vi "日志信息主动发送(子VI).vi"(10 "是否正在查询数据":bool, 11 "查询数据发送时间节点":string) -> ()   [LabVIEW 2016, in "数据传输系统.lvlib"]
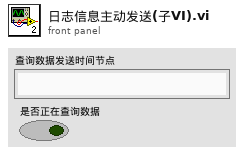
[diagram p1: front panel]
types:
  T1 = typedef "LVDateTimeRec.ctl" = cluster{"秒数的小数部分":dbl, "秒":i32, "分":i32, "时":i32, "日":i32, "月":i32, "年":i32, "天数（周）":i32, "天数（年）":i32, "DST":i32}
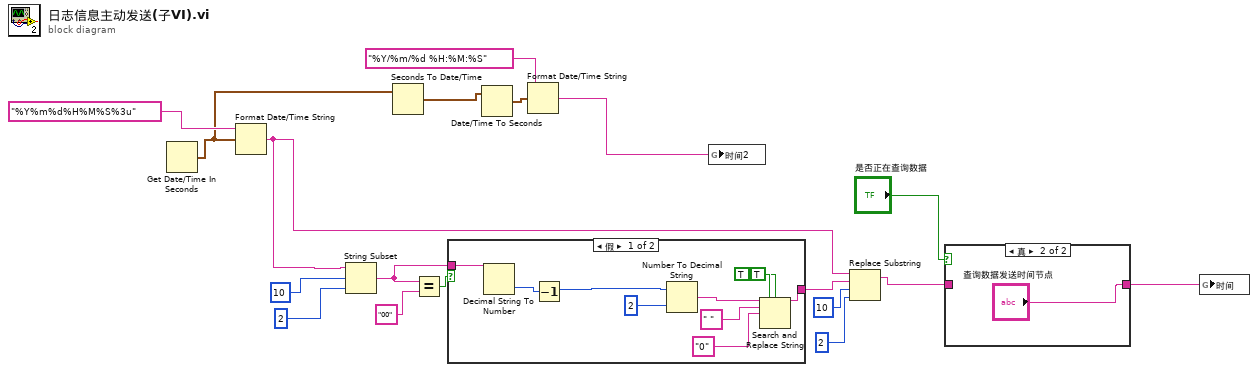
[diagram p0: block diagram]
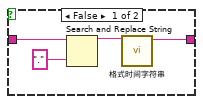
[diagram p2: hidden frame]
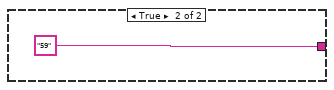
[diagram p3: hidden frame]
diagram:
  n1 = Get Date/Time In Seconds() -> (seconds since 1Jan1904=w2:timestamp)
  n2 = Format Date/Time String(time format string (%c)="%Y%m%d%H%M%S%3u" ("时间格式字符串(%c)"), seconds (now)=w2) -> (date/time string=w7:string)  [unwired: 1 in]
  n3 = String Subset(string=w7, offset (0)=10 ("偏移量(0)"), length (rest)=2 ("长度（子字符串长度）")) -> (substring=w15:string)
  n4 = Seconds To Date/Time(time stamp (now)=w2) -> (date time rec=w3:T1)  [unwired: 1 in]
  n5 = Equal?(x=w15, y="00") -> (x = y?=w14:bool)
  n6 = case shown="假" w14 {
    tunnel: w15 -> [w28 _]
    tunnel: [w20 "59" ("y")] -> w16
    frame False {
      n7 = Decimal String To Number(string=w28) -> (number=w27:i32)  [unwired: 2 in, 1 out]
      n8 = Decrement(x=w27) -> (x-1=w21:i32)
      n9 = Number To Decimal String(number=w21, width (-)=i16 2 ("宽度(-)")) -> (decimal integer string=w23:string)
      n10 = Search and Replace String(replace all?=TRUE ("替换全部？(F)"), case sensitive?=TRUE ("忽略大小写？(F)"), input string=w23, search string=" " ("搜索字符串"), replace string="0" ("替换字符串(\"\")")) -> (result string=w20:string)  [unwired: 3 in, 3 out]
    }
    frame True {
    }
  }
  n11 = Date/Time To Seconds(2:w3) -> (0:w5:timestamp)  [unwired: 1 in]
  n12 = Format Date/Time String(time format string (%c)="%Y/%m/%d %H:%M:%S" ("时间格式字符串(%c)"), seconds (now)=w5) -> (date/time string=w1:string)  [unwired: 1 in]
  n13 = global write "全局 时间2.vi" "时间2"(w1) -> ()
  n14 = Replace Substring(2:2 ("长度（子字符串长度）"), 3:10 ("偏移量(0)"), 4:w16, 5:w7) -> (1:w8:string)  [unwired: 1 out]
  n15 = case shown="真" "是否正在查询数据" {
    tunnel: [w31 "查询数据发送时间节点"] -> w9
    tunnel: w8 -> [w30 _]
    frame False {
      n16 = Search and Replace String(input string=w30, search string="." ("搜索字符串")) -> (result string=w32:string)  [unwired: 6 in, 3 out]
      n17 = call "格式时间字符串.vi"("字符串"=w32) -> ("连接的字符串"=w31:string)  [unwired: 10 in]
    }
    frame True {
    }
  }
  n18 = global write "全局 水样时间.vi" "时间"(w9) -> ()
